vi "RVC Lane change (Subsystem).vi"() -> ()   [LabVIEW 2013]
uses:
  SIM Bicycle.vi
  <vilib>/Simulation/Implementation/Shared/SIMSCR Execution Mode.ctl
  <vilib>/Simulation/Scripting/Companion Diagram/SimConfigNode/SimParams.ctl
  <vilib>/Simulation/Scripting/Companion Diagram/SimConfigNode/_simSolvers.ctl
  <vilib>/Simulation/Param Hierarchy/Typedefs/SIMPH Param Control Actions.ctl
  <vilib>/Simulation/Implementation/Shared/NILVSim_ParamChanged.vi
  <vilib>/Simulation/Implementation/Shared/NILVSIM_BeginStep.vi
  <vilib>/Simulation/Utility/Implementation/SIM Time.vi
  <vilib>/Simulation/LookUpTables/Implementation/NILVSim LUT 1D.llb/SIM LUT 1D (scalar).vi
  <vilib>/Simulation/SignalDisplay/Implementation/NILVSim Time Waveform.llb/SIM Time Waveform (scalar).vi
  <vilib>/Simulation/SignalDisplay/Implementation/NILVSim Buffer XY Graph.llb/SIM Buffer XY Graph (scalar).vi
  <vilib>/Simulation/Implementation/Shared/NILVSim_Manager.vi
  <vilib>/Simulation/Implementation/Shared/NILVSim_FinalizeModel.vi
  <vilib>/Simulation/SignalDisplay/Implementation/NILVSim Buffer XY Graph.llb/NILVSim Buffer XY Graph (core).vi
  <vilib>/Simulation/Implementation/Shared/SIM manage modulo counter.vi
  <vilib>/Simulation/Implementation/Shared/SIM Circular Buffer.llb/SIM CircBuf remove oldest.vi
  <vilib>/Simulation/Implementation/Shared/SIM Circular Buffer.llb/SIM circular buffer insert.vi
  <vilib>/Simulation/Implementation/Shared/SIM Unbundle Sim Info.vi
  <vilib>/Utility/error.llb/Clear Errors.vi
  <vilib>/Simulation/Implementation/Shared/NILVSim_GetModelError.vi
  <vilib>/Simulation/Implementation/Shared/SIM SimErrorHandler.vi
  <vilib>/Simulation/Implementation/Shared/SIM Bundle Sim Info.vi
  <vilib>/Simulation/Implementation/Shared/SIMSH Read Queue.vi
  <vilib>/Simulation/Implementation/Shared/NILVSim_Initialize.vi
  <vilib>/Simulation/Utility/Implementation/NILVSim Get Time and IsAcceptedStep.vi
  <vilib>/Simulation/Implementation/Shared/SIM Circular Buffer.llb/SIM circular buffer ordered array.vi
  <vilib>/Simulation/Implementation/Shared/SIM Circular Buffer.llb/SIM circular buffer create.vi
  <vilib>/Simulation/Scripting/Companion Diagram/SimConfigNode/SimDog.xnode
  <vilib>/Simulation/Implementation/XNodeFramework/SimXNode/SimX.xnode
  <vilib>/Simulation/Implementation/Shared/NI_SIM_Implementation.lvlib
panel:
  out "alpha":waveform(dbl)(graph)
  out "theta":waveform(dbl)(graph)
  out "XY Graph":cluster{dbl, dbl}[](graph)
  out "y":waveform(dbl)(graph)
  in  "velocity":dbl(slide)=1.0 scale=0.0..10.0
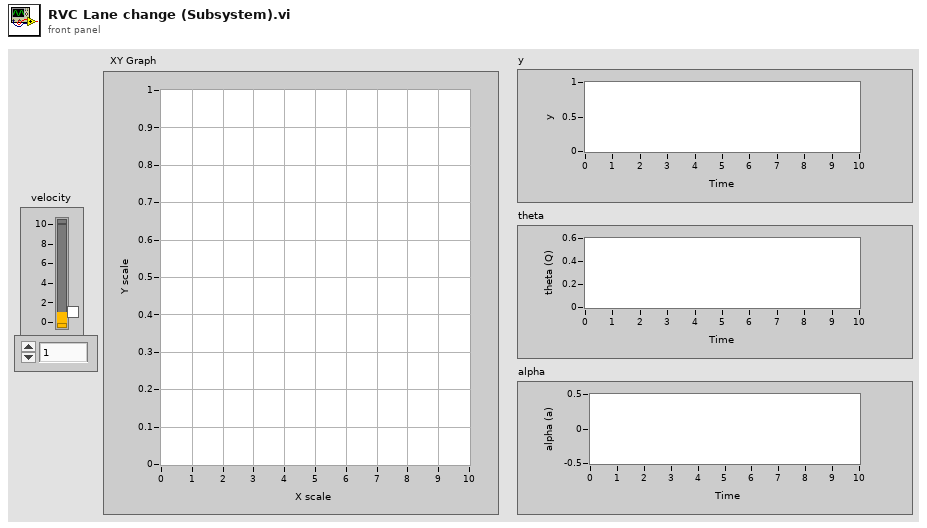
[diagram p1: front panel]
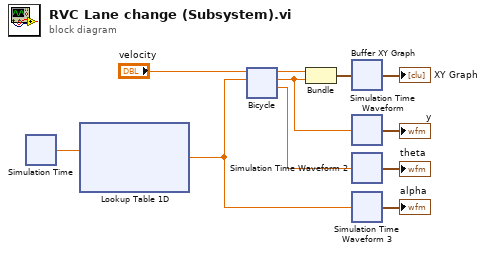
[diagram p0: block diagram]
diagram:
  n1 = xnode "Simulation Time"() -> ("simulation time"=w10:dbl)  [unwired: 2 in]
  n2 = xnode "Lookup Table 1D"("X Val"=w10) -> ("Result"=w4:dbl)  [unwired: 5 in]
  n3 = xnode "Bicycle"("gamma"=w4, "v"="velocity") -> ("theta"=w1:dbl, "y"=w5:dbl, "x"=w8:dbl)  [unwired: 3 in, 4 out]
  n4 = Bundle ("Bundle 2")("x"=w8, "y"=w5) -> (w7:cluster{"x":dbl, "y":dbl})  [unwired: 1 in]
  n5 = xnode ("Buffer XY Graph")("Value"=w7) -> ("XY Graph"=→"XY Graph":cluster{"X":dbl, "Y":dbl}[])  [unwired: 4 in]
  n6 = xnode ("Simulation Time Waveform")("Value"=w5) -> ("Waveform Chart"=→"y":waveform(dbl))  [unwired: 1 in]
  n7 = xnode ("Simulation Time Waveform 2")("Value"=w1) -> ("Waveform Chart"=→"theta":waveform(dbl))  [unwired: 1 in]
  n8 = xnode ("Simulation Time Waveform 3")("Value"=w4) -> ("Waveform Chart"=→"alpha":waveform(dbl))  [unwired: 1 in]
